vi "Keyence.Main-GetTablePosition.vi"(8 "error in (no error)":errorcluster, 9 "Force (F)":bool, 11 "ScannerSlot in":i32) -> (0 "error out":errorcluster, 2 "TestStatus":T1[](array[typedef]), 3 "ScannerSlot out":i32)   [LabVIEW 2016]
uses:
  Keyence.Data.Status.ctl
  Keyence.Data.Status.State.ctl
  LowLevel/Keyence.CodeDetails.ctl
  Sequence/Sequence.Test.Status.ctl
  Sequence/Sequence.Slot.StatusData.ctl
  Sequence/Sequence.Test.Unload.Status.ctl
  Sequence/Sequence.Prod.StatusData.ctl
  Sequence/Sequence.Step.Status.ctl
  Sequence/Sequence.Test.BreakReason.ctl
  tools/Translator/Translator.Message.ctl
  tools/EventLog/EventLog.EventSource.ctl
  tools/EventLog/EventLog.CreateError(single).vi
panel:
  out "data":T7
  out "Final status":T8={"State"=enum."Init", "Ref"=refnum, "Bank"=0, "Version"="", "Model"="", "EndTS"=timestamp(0 s since 1904-01-01), "ImgPath"=path "", "Tuned"=FALSE}
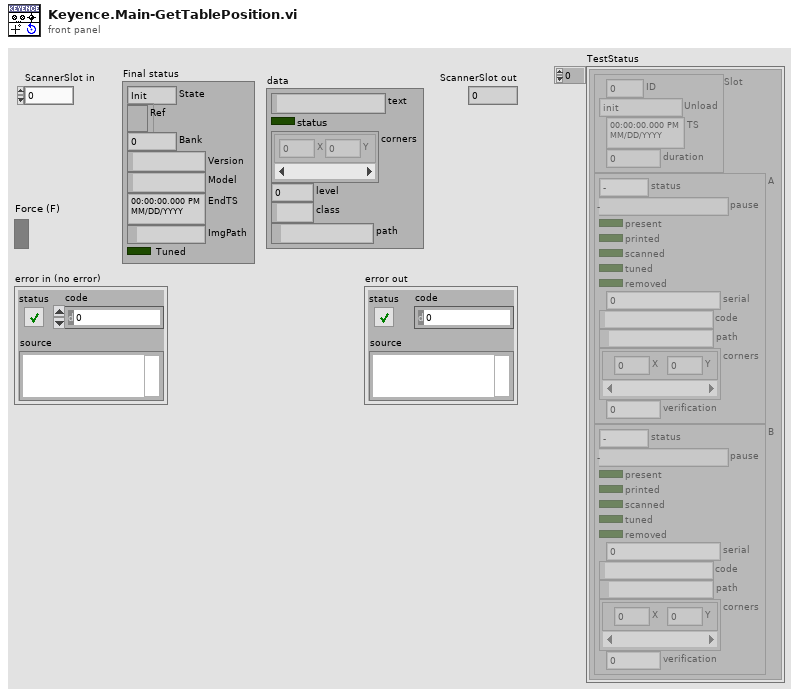
[diagram p1: front panel]
types:
  T1 = typedef "Sequence.Test.Status.ctl" = cluster{"Slot":T2, "A":T4, "B":T4}
  T2 = typedef "Sequence.Slot.StatusData.ctl" = cluster{"ID":i32, "Unload":T3, "TS":timestamp, "duration":u32}
  T3 = typedef "Sequence.Test.Unload.Status.ctl" = enum16{"init", "check NOK", "check OK", "wait on NOK", "wait on OK", "wait on Unload", "done"}
  T4 = typedef "Sequence.Prod.StatusData.ctl" = cluster{"status":T5, "pause":T6, "present":bool, "printed":bool, "scanned":bool, "tuned":bool, "removed":bool, "serial":i32, "code":string, "path":path, "corners":cluster{"X":i32, "Y":i32}[], "verification":u8}
  T5 = typedef "Sequence.Step.Status.ctl" = enum16{"-", "Pending", "Running", "Skipped", "Passed", "Failed", "Done", "Error", "Aborted", "Stopped"}
  T6 = typedef "Sequence.Test.BreakReason.ctl" = enum16{"-", "NOK container", "OK container", "Rev empty", "Rev missing", "Rev wrong", "Fork missing", "Fork wrong", "NOK limit", "Unload failure", "Single slot", "Part done", "Err: Prod move work", "Err: Prod move home", "Err: Prod lift work", "Err: Prod lift home", "Err: Prod Arm Work", "Err: Prod Arm NOK", "Err: Prod Arm OK", "Err: Prod NOK suck", "Err: Prod NOK drop", "Err: Prod OK missing", "Err: Prod OK suck", "Err: Prod OK drop"}
  T7 = typedef "Keyence.CodeDetails.ctl" = cluster{"text":string, "status":bool, "corners":cluster{"X":i32, "Y":i32}[], "level":u8, "class":string, "path":path}
  T8 = typedef "Keyence.Data.Status.ctl" = cluster{"State":T9, "Ref":refnum<k5>, "Bank":u8, "Version":string, "Model":string, "EndTS":timestamp, "ImgPath":path, "Tuned":bool}
  T9 = typedef "Keyence.Data.Status.State.ctl" = enum16{"First", "Init", "Reset", "Idle", "Scan", "Tune"}
  T10 = typedef "EventLog.EventSource.ctl" = enum16{"All", "Gui", "Ref", "File", "Arch", "Seq", "CPX", "DB", "Laser", "Scan.P", "Scan.O"}
  T11 = typedef "Translator.Message.ctl" = enum16{"-", "Event confirmed", "Log out", "Log in", "Shutdown", "Cancel", "Start", "Begin time", "End time", "Duration", "Service Mode", "Ignore Results", "Serial Format", "On", "Off", "OK", "NOK", "NOK %s", "Home", "Work", "Close", "Open", "In progress...", "Missing", "Empty", "Hardware failure", "Initial", "Default", "Total", "Out of range", "Free disk space is below 1GB - contact technician", "Error %d >> %s", "Error %d >> %s >> %s", "Msg %d >> %s", "Laser msg %d %s", "Laser cmd error %s %d", "Laser cmd failed %s", "Laser cmd warning %s", "Laser disconnected", "Laser status %s", "Laser already started", "Laser job unkonwn %s", "Laser job missing %s", "Laser job select failure %s", "Unable to start laser printing (%s)", "Unable to stop laser printing (%s)", "Laser marking aborted", "Laser marking timeout", "Unable to reset Laser Interlock (%s)", "Unable to trigger Laser. Laser not ready (%s)", "Laser job '%s' coordinates not configured", "Starting %s", "Quitting %s", "Configured", "Initializing", "Quitting", "Loading", "Loaded %d results", "Loaded %d events", "Running", "Stopped", "Summary", "Laser", "Do you want to continue?", "Do you want to delete the configuration?", "The configuration is being used by an order. Unable to delete!", "Press confirm button", "Station is not based. Do you want to exit?", "Station requires changeover. Do you want to run the test?", "Test options are not set as default. Do you want to continue?", "Formatting of WabcoNo is disabled. Do you want to continue?", "Product not detected. Do you want to continue?", "Product scan failed. Do you want to continue?", "Calibration", "Log out?", "System", "All", "IDLE", "Translating...%s", "Not found", "Alarm %s", "Run", "Skip", "Abort", "Repeat", "Please wait...", "Database disconnected", "Database disconnected - changeover disabled!", "Login to database successful", "Login to database failed: %d; %s", "Unable to check the product status of reference %d - database disconnected", "Unable to set the product status of reference %d - database disconnected", "Variant file backup %s", "Read variant (%s)", "Result", "Station armed!", "Station requires changeover!", "Select reference number...", "EMERGENCY BUTTON - press Control button", "EMERGENCY DOOR - press Control button", "Resetting Emergency...", "Unable to reset safety circuit - Emergency Button pressed", "Unable to reset safety circuit - Emergency Side Door open", "Station not based", "Station based", "Station not empty", "Station basing...", "No order", "Press Start to begin new order", "Scanning new order", "Order NOK. Correct or scan again", "Order OK. Press Accept", "Order ready", "Revolver incorrect", "Fork incorrect", "Revolver missing", "Revolver empty", "Container missing", "Offline results", "Offline statistics", "Updating statistics %.1f %%", "DMC Configurator", "Door open", "Close the front door", "Press start button", "Done. Open the front door", "Running...", "Running...%.1f %%", "Pause %s", "Pause %s. NOK container missing", "Pause %s. OK container missing", "Pause %s. Revolver empty", "Pause %s. Revolver missing", "Pause %s. Revolver incorrect", "Pause %s. Fork missing", "Pause %s. Fork incorrect", "Pause %s. Too many failures", "Pause %s. Unloading failure", "Pause %s. One slot is not working", "Pause %s. Part order is done. Empty OK container", "Pause %s. Unable to move product to slot", "Pause %s. Unable to move back product pusher", "Pause %s. Unable to lift product", "Pause %s. Unable to move back product lifter", "Pause %s. Unable to move product arm to Work", "Pause %s. Unable to move product arm to NOK", "Pause %s. Unable to move product arm to OK", "Pause %s. Unable to unsuck the NOK product", "Pause %s. Unable to drop the NOK product", "Pause %s. Product OK missing", "Pause %s. Unable to unsuck the OK product", "Pause %s. Unable to drop the OK product", "Stopping...", "File '%s' is missing", "File '%s' is broken", "File '%s' is running", "Log file started (%s)", "Log file ended (%s)", "Log file stopped (%s)", "Log file ignored (%s)", "Log file exported (%s)", "Log file export failed (%s)", "Wrong serial number in log file", "Wrong reference number in log file", "Test steps are missing", "%s = %.3f", "Process param '%s' not found in DB", "Process param '%s' wrong order", "Process param '%s' value %.3f out of limits (%.3f; %.3f)", "Step%d param '%s' not found in DB", "Step%d param '%s' wrong order", "Step%d param '%s' value %.3f out of limits (%.3f; %.3f)", "Step%d EV '%s' not found in DB", "Step%d EV '%s' wrong order", "\"%s\" not found in DB", "\"%s\" wrong order", "\"%s\" value %.3f out of limits (%.3f; %.3f)", "\"%s\" not found in software", "Process init (%s)", "Process started", "Process restarted", "Process run", "Process done", "Process done - remove OK container", "Process aborted", "Process aborted at work", "Process aborted at home", "Process error", "Process error at home", "Process error at work", "Process close", "Process pause", "Process continue", "Process door open", "Process door close", "Process pause at slot %s due to %s", "Select plate from the order to process", "Do you want to start the process?", "Do you want to continue the process?", "There is unfinished order. Do you want to put the new order?", "Product %s %d OK", "Product %s %d NOK", "Unable to unload the slot %s. Product missing in the slot", "Unable to unload the slot %s. Product already in the arm", "Unable to accept the product as OK. Product missing in slot %s", "Unable to accept the product as OK. Product could not drop into the container at slot %s", "Unable to accept the product as NOK. Product could not drop into the container at slot %s", "Scan failed. Error %s", "Scan failed. Scanner disconnected", "Scan failed. Wrong Wabco number %d, limit (%d,%d)", "Scan failed. Wrong serial number %d, limit (%d,%d)", "Scan failed. Wrong date %d, limit (%d,%d)", "Scan failed. Wrong product wabco number %d (expected %d)", "Scan failed. Wrong product serial number %d (expected > 0)", "Scan OK %s", "Scan failed. Unable to determine table position (%s)", "Scan failed. Timeout", "Tune failed. Scanner disconnected", "Tune failed. Timeout", "%s = %d", "%s = %d->%d", "Unable to set %s = %.2f - Air Pressure Inside off", "Unable to set digital output '%s' = %d", "Unable to activate air pressure inside - timeout", "Unable to activate air pressure inside - aborted", "Unable to switch on Air Main Valve - Air Pressure Inlet off", "Unable to switch on Air Main Valve - Door open", "Unable to switch off Air Main Valve - timeout", "Unable to switch off Air Main Valve - aborted", "Unable to rotate Table - timeout", "Unable to rotate Table - aborted", "Unable to rotate Table - Product Move not in Home position", "Unable to rotate Table - Air Pressure Inside off", "Unable to rotate Table - Product Lift A not in Home position", "Unable to rotate Table - Product Lift B not in Home position", "Unable to rotate Table - unlock before movement timeout", "Unable to rotate Table - lock after movement timeout", "Unable to move Table Lock to %s position - timeout", "Unable to move Table Lock to %s position - aborted", "Unable to move Table Lock to %s position - Air Pressure Inside off", "Unable to move Table Lock to %s position - Table not in position", "Unable to move Product Lift A to %s position - timeout", "Unable to move Product Lift B to %s position - timeout", "Unable to move Product Lift A to %s position - aborted", "Unable to move Product Lift B to %s position - aborted", "Unable to move Product Lift A to %s position - Air Pressure Inside off", "Unable to move Product Lift B to %s position - Air Pressure Inside off", "Unable to move Product Lift A to %s position - Table not locked", "Unable to move Product Lift B to %s position - Table not locked", "Unable to move Product Lift A to %s position - Product Arm not in Work position", "Unable to move Product Lift B to %s position - Product Arm not in Work position", "Unable to set Product Suction Gripper %s to %s - timeout", "Unable to set Product Suction Gripper %s to %s - aborted", "Unable to set Product Suction Gripper %s to %s - Air Pressure Inside off", "Unable to set Product Suction Gripper %s to %s - Table slot unkown", "Unable to move Product Arm to %s position - timeout", "Unable to move Product Arm to %s position - aborted", "Unable to move Product Arm to %s position - Air Pressure Inside off", "Unable to move Product Arm to %s position - Product Lift A not in Home position", "Unable to move Product Arm to %s position - Product Lift B not in Home position", "Unable to move Product to %s position - timeout", "Unable to move Product to %s position - aborted", "Unable to move Product to %s position - Air Pressure Inside off", "Unable to move Product to %s position - Table not in position"}
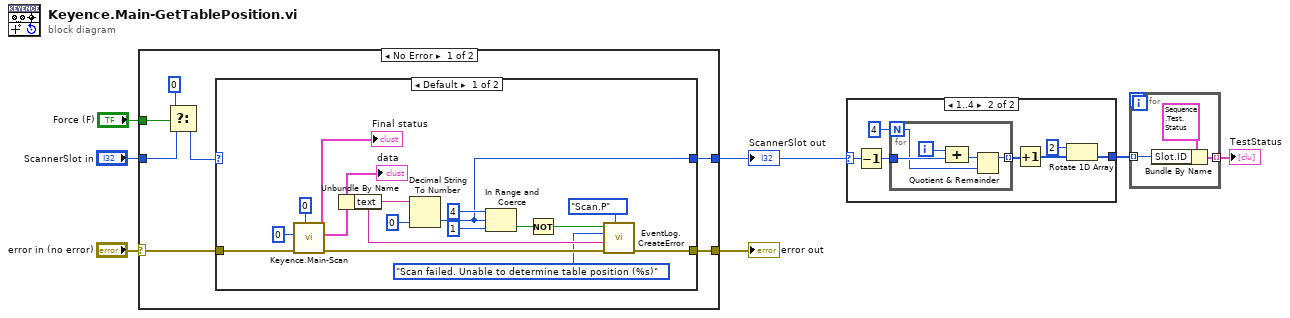
[diagram p0: block diagram]
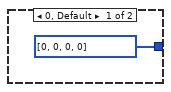
[diagram p2: hidden frame]
diagram:
  n1 = case shown="No Error" "error in (no error)" {
    selector: "error in (no error)" -> [w12 w33]
    tunnel: [w14 w33] -> w7
    tunnel: "ScannerSlot in" -> [w10 w34]
    tunnel: [w13 w34] -> w3
    tunnel: "Force (F)" -> [w11 _]
    frame No Error {
      n2 = Select(t=0, s=w11, f=w10) -> (s? t:f=w8:i32)
      n3 = case shown="Default" w8 {
        selector: w8 -> [_ w32]
        tunnel: [w30 w31] -> w14
        tunnel: w12 -> [w29 w31]
        tunnel: [w17 w32] -> w13
        frame Default {
          n4 = call "Keyence.Main-Scan.vi"("Idx"=0, "error in"=w29, "Bank"=u8 0) -> ("error out"=w24:errorcluster, "Code"=w15:T7, "Final status"=→"Final status":T8)  [unwired: 6 in]
          "data" <- w15
          n5 = Unbundle By Name(w15) -> ("text"=w22:string)
          n6 = Decimal String To Number(string=w22, default (0L)=0 ("default (0 I32)")) -> (number=w17:i32)  [unwired: 1 in, 1 out]
          n7 = In Range and Coerce(upper limit=4, x=w17, lower limit=1) -> (In Range?=w19:bool)  [unwired: 1 out]
          n8 = Not(x=w19) -> (.not. x?=w21:bool)
          n9 = call-poly "EventLog.CreateError.vi"("Source (All)"=EventLog.EventSource."Scan.P", "error in"=w24, "arg"=w22, "msg"=Translator.Message."Scan failed. Unable to determine table position (%s)", "create (T)"=w21) -> ("error out"=w30:errorcluster)  [unwired: 6 in]
        }
        frame 1..4 {
        }
      }
    }
    frame Error {
    }
  }
  "error out" <- w7
  "ScannerSlot out" <- w3
  n10 = case shown="1..4" w3 {
    selector: w3 -> [_ w36]
    tunnel: [i32[] [0, 0, 0, 0] w39] -> w4
    frame 0, Default {
    }
    frame 1..4 {
      n11 = Decrement(x=w36) -> (x-1=w42:i32)
      n12 = for {
        N: 4 -> [w44]
        tunnel: w42 -> [w46]
        tunnel: [w43] -> w41 mode=indexing
        i -> [w47]
        n13 = Compound Arithmetic op=ADD(w47, w46) -> (w45:i32)
        n14 = Quotient & Remainder(x=w45, y=w44) -> (x-y*floor(x/y)=w43:i32)  [unwired: 1 out]
      }
      n15 = Increment(x=w41) -> (x+1=w40:i32[])
      n16 = Rotate 1D Array(1:w40, 2:2 ("n")) -> (0:w39:i32[])
    }
  }
  n17 = for {
    tunnel: [w49] -> w2 mode=indexing
    tunnel: w4 -> [w48] mode=indexing
    n18 = Bundle By Name(cluster=T1 {"Slot"={"ID"=0, "Unload"=enum."init", "TS"=timestamp(0 s since 1904-01-01), "duration"=0}, "A"={"status"=enum."-", "pause"=enum."-", "present"=FALSE, "printed"=FALSE, "scanned"=FALSE, "tuned"=FALSE, "removed"=FALSE, "serial"=0, "code"="", "path"=path "", "corners"=[], "verification"=0}, "B"={"status"=enum."-", "pause"=enum."-", "present"=FALSE, "printed"=FALSE, "scanned"=FALSE, "tuned"=FALSE, "removed"=FALSE, "serial"=0, "code"="", "path"=path "", "corners"=[], "verification"=0}} ("Data in"), "Slot.ID"=w48) -> (w49:T1)
  }
  "TestStatus" <- w2
